vi "getChildEvents.vi"(8 "error in (no error)":errorcluster, 11 "cameraSettingsEventManager in":refnum<class "cameraSettingsEventManager.lvclass">) -> (0 "error out":errorcluster, 2 "cameraSettingsEventsRef":T1, 3 "cameraSettingsEventManager out":refnum<class "cameraSettingsEventManager.lvclass">)   [LabVIEW 2009, in "Tools.lvlib" / "Settings.lvlib" / "cameraSettingsEventManager.lvclass"]
uses:
  cameraSettingsEventManager.lvclass
  Tools/Settings.lvlib
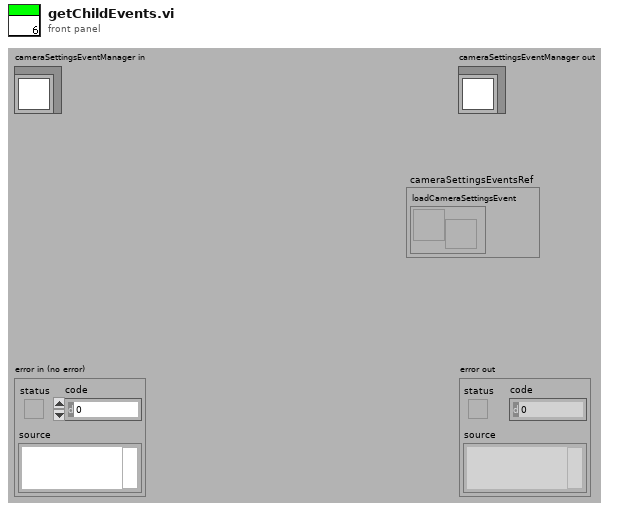
[diagram p1: front panel]
types:
  T1 = cluster{"loadCameraSettingsEvent":refnum<user-event>}
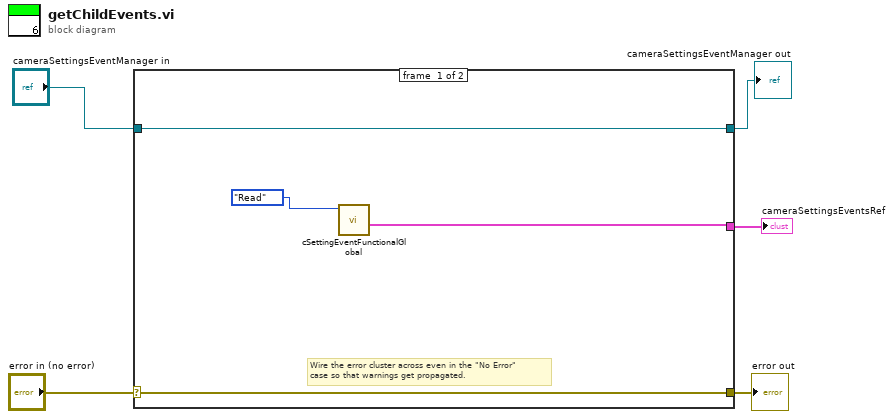
[diagram p0: block diagram]
diagram:
  n1 = case shown="No Error" "error in (no error)" {
    selector: "error in (no error)" -> [w8 w11]
    tunnel: [w8 w11] -> w4
    tunnel: [w9 w10] -> w2
    tunnel: "cameraSettingsEventManager in" -> [w9 w10]
    tunnel: [w6 _] -> w1
    frame #0 {
      # "Wire the error cluster across even in the \"No Error\"\ncase so that warnings get propagated."
      n2 = call "cSettingEventFunctionalGlobal.vi"("Action"=enum16{"Write", "Read"}."Read") -> ("cameraSettingsEventsRef"=w6:T1)  [unwired: 10 in]
    }
    frame #1 {
    }
  }
  "error out" <- w4
  "cameraSettingsEventManager out" <- w2
  "cameraSettingsEventsRef" <- w1
